vi "Shutdown.vi"(8 "error in":errorcluster, 11 "nCRD in":refnum<class "gCRD.lvclass">) -> (0 "error out":errorcluster, 3 "nCRD out":refnum<class "gCRD.lvclass">)   [LabVIEW 2017, in "gCRDS.lvlib" / "gCRD.lvclass"]
uses:
  gCRD.lvclass
  Session/Raw FPGA/FPGA Session.lvclass
  C:/Program Files (x86)/National Instruments/LabVIEW 2017/vi.lib/MSR Consulting, LLC/General Reuse/Session APIs/_Session Fwk/Session - Root.lvclass
  gCRD.lvclass/gCRD.ctl
  <vilib>/MSR Consulting, LLC/General Reuse/CRDS/Main/CRDS.lvclass
  <vilib>/MSR Consulting, LLC/General Reuse/Session APIs/_Session Fwk/Session - Root.lvclass
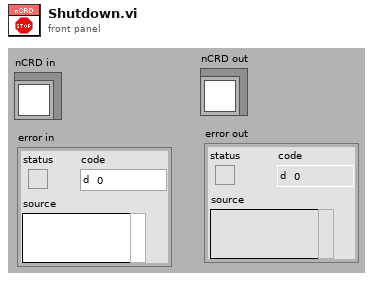
[diagram p1: front panel]
types:
  T1 = typedef "Session - Root.lvclass/Session Handle.ctl" = refnum<data-value>
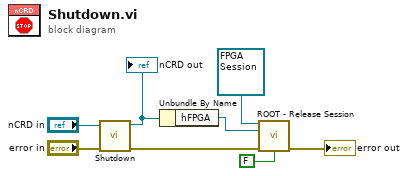
[diagram p0: block diagram]
diagram:
  n1 = call-parent "Shutdown.vi"("error in"="error in", "Instrument in"="nCRD in") -> ("error out"=w1:errorcluster, "Instrument out"=w6:refnum<class "gCRD.lvclass">)  [unwired: 8 in]
  "nCRD out" <- w6
  n2 = Unbundle By Name(w6) -> ("hFPGA"=w5:T1)
  n3 = call <vilib>:"ROOT - Release Session.vi"("OBJ - Session in"=refnum<class "FPGA Session.lvclass"> refnum ("FPGA Session"), "Session Handle in"=w5, "error in (no error)"=w1, "force destroy? (F)"=FALSE) -> ("error out"=→"error out":errorcluster)  [unwired: 10 in, 1 out]
